vi "name tables.vi"(7 "2D?":bool, 8 "error in":errorcluster, 9 "Z Slice":string, 10 "ROI":string, 11 "path folder in":path) -> (0 "error out":errorcluster, 3 "path file out":path)   [LabVIEW 2023]
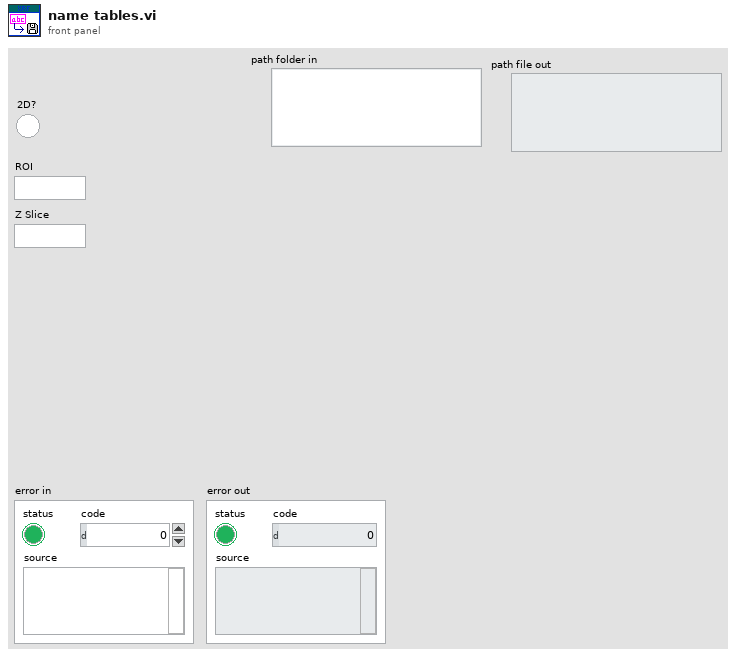
[diagram p1: front panel]
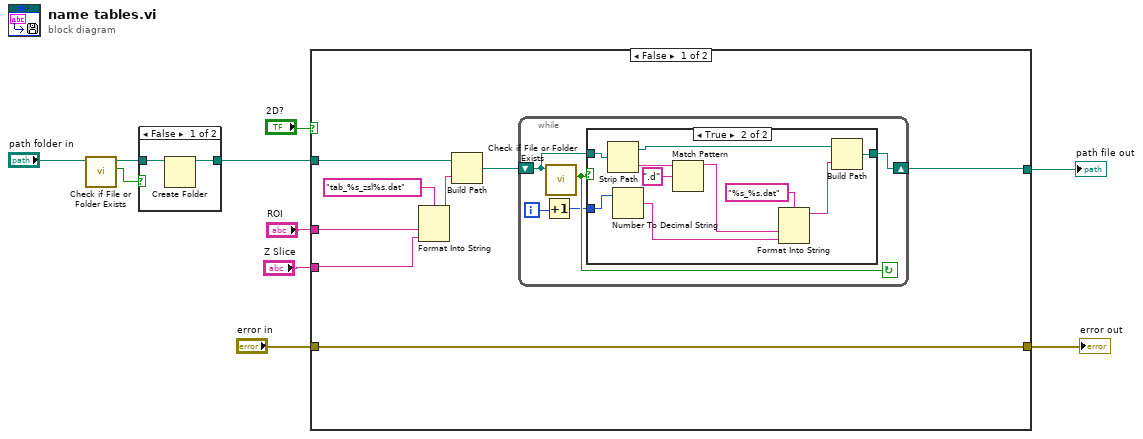
[diagram p0: block diagram]
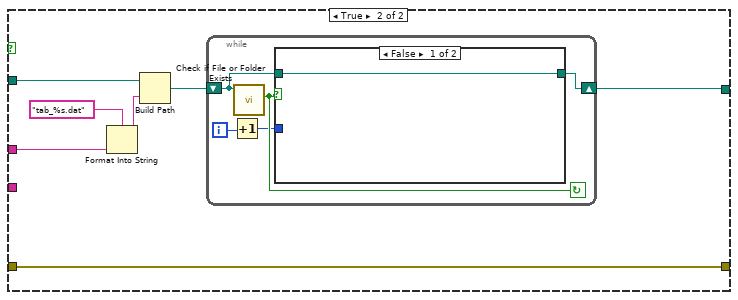
[diagram p4: hidden frame]
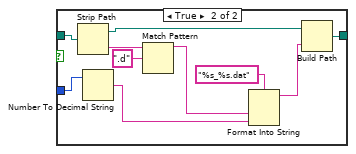
[diagram p5: hidden frame]
diagram:
  n1 = call <vilib>:"Check if File or Folder Exists.vi"("path"="path folder in") -> ("file or folder exists?"=w4:bool, "dup path"=w3:path)  [unwired: 8 in, 1 out]
  n2 = case shown="False" w4 {
    tunnel: w3 -> [w12 w13]
    tunnel: [w11 w13] -> w2
    frame False {
      n3 = Create Folder(path (use dialog)=w12) -> (created path=w11:path)  [unwired: 2 in, 2 out]
    }
    frame True {
    }
  }
  n4 = case shown="False" "2D?" {
    tunnel: [w21 w44] -> w10
    tunnel: "error in" -> [w21 w44]
    tunnel: w2 -> [w17 w43]
    tunnel: "ROI" -> [w16 w40]
    tunnel: "Z Slice" -> [w15 _]
    tunnel: [w14 w38] -> w5
    frame False {
      n5 = Format Into String(format string="tab_%s_zsl%s.dat", w16, w15) -> (resulting string=w19:string)  [unwired: 2 in, 1 out]
      n6 = Build Path(base path=w17, name or relative path=w19) -> (appended path=w18:path)
      n7 = while {
        shift-right: [w25] -> w14
        shift-left: w18 -> [w26]
        i -> [w23]
        stop <- w24 continue-if-true
        n8 = Increment(x=w23) -> (x+1=w22:i32)
        n9 = call <vilib>:"Check if File or Folder Exists.vi"("path"=w26) -> ("file or folder exists?"=w24:bool)  [unwired: 8 in, 2 out]
        n10 = case shown="True" w24 {
          tunnel: w26 -> [w27 w36]
          tunnel: [w27 w35] -> w25
          tunnel: w22 -> [_ w37]
          frame False {
          }
          frame True {
            n11 = Strip Path(path=w36) -> (stripped path=w34:path, name=w30:string)
            n12 = Number To Decimal String(number=w37) -> (decimal integer string=w31:string)  [unwired: 1 in]
            n13 = Match Pattern(string=w30, regular expression=".d") -> (before substring=w28:string)  [unwired: 1 in, 3 out]
            n14 = Format Into String(format string="%s_%s.dat", w28, w31) -> (resulting string=w32:string)  [unwired: 2 in, 1 out]
            n15 = Build Path(base path=w34, name or relative path=w32) -> (appended path=w35:path)
          }
        }
      }
    }
    frame True {
      n16 = Format Into String(format string="tab_%s.dat", w40) -> (resulting string=w41:string)  [unwired: 2 in, 1 out]
      n17 = Build Path(base path=w43, name or relative path=w41) -> (appended path=w39:path)
      n18 = while {
        shift-right: [w48] -> w38
        shift-left: w39 -> [w49]
        i -> [w46]
        stop <- w47 continue-if-true
        n19 = Increment(x=w46) -> (x+1=w45:i32)
        n20 = call <vilib>:"Check if File or Folder Exists.vi"("path"=w49) -> ("file or folder exists?"=w47:bool)  [unwired: 8 in, 2 out]
        n21 = case shown="False" w47 {
          tunnel: w49 -> [w50 w59]
          tunnel: [w50 w58] -> w48
          tunnel: w45 -> [_ w60]
          frame False {
          }
          frame True {
            n22 = Strip Path(path=w59) -> (stripped path=w57:path, name=w53:string)
            n23 = Number To Decimal String(number=w60) -> (decimal integer string=w54:string)  [unwired: 1 in]
            n24 = Match Pattern(string=w53, regular expression=".d") -> (before substring=w51:string)  [unwired: 1 in, 3 out]
            n25 = Format Into String(format string="%s_%s.dat", w51, w54) -> (resulting string=w55:string)  [unwired: 2 in, 1 out]
            n26 = Build Path(base path=w57, name or relative path=w55) -> (appended path=w58:path)
          }
        }
      }
    }
  }
  "error out" <- w10
  "path file out" <- w5
